vi "Playground_Variant Attributes to Cluster.vi"() -> ()   [LabVIEW 2019]
uses:
  subVIs/typedefs/Schedule Types/Schedule--Ramp.ctl
  Classes/Settings/ObjectSettings/ObjectSettings.lvclass
panel:
  out "Array":variant[](array[variant])
  out "x/y":dbl
  # "Read"
  # "JDP: 4.65363E-5"
  # "JKI: 0.0002399"
  # "Write"
  # "JDP: 3.40146E-5\nJKI: 8.64174E-5"
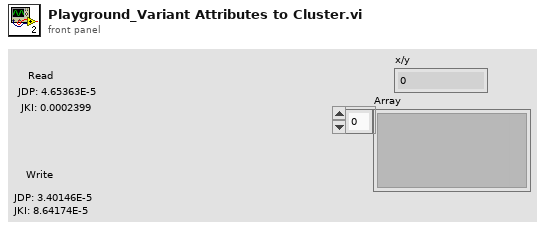
[diagram p1: front panel]
types:
  T1 = typedef "Schedule--Ramp.ctl" = cluster{"Start":dbl, "End":dbl}
  T2 = cluster{"Attribute 1":bool, "Attribute 2":string, "Attribute 3":string}
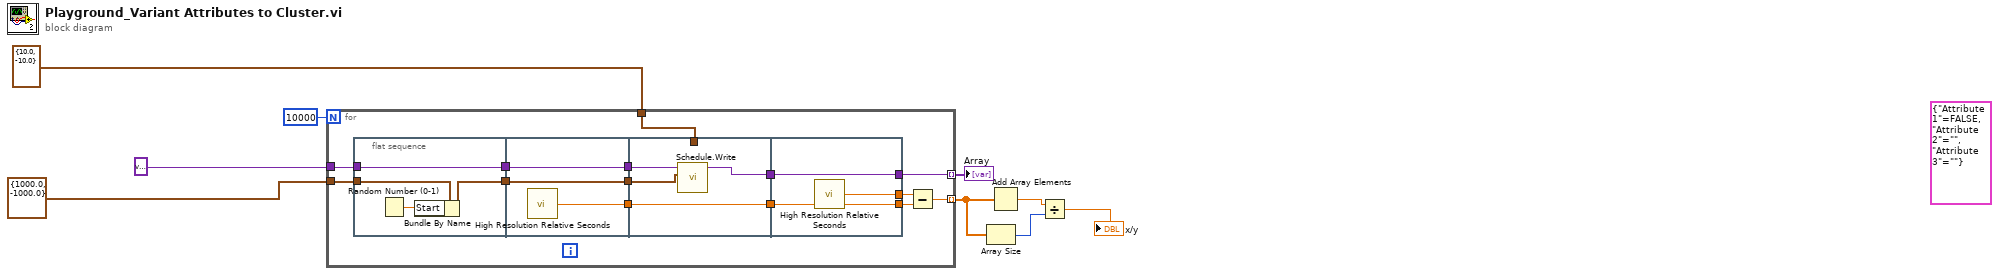
[diagram p0: block diagram]
diagram:
  (unwired) T2 {"Attribute 1"=FALSE, "Attribute 2"="", "Attribute 3"=""}
  n1 = for {
    N: 10000 -> [_]
    tunnel: T1 {"Start"=10.0, "End"=-10.0} ("Ramp") -> [w21]
    tunnel: variant ("LUT In") -> [w23]
    tunnel: [w22] -> w1 mode=indexing
    tunnel: [w14] -> w7 mode=indexing
    tunnel: T1 {"Start"=1000.0, "End"=-1000.0} ("Ramp") -> [w11]
    n2 = flat-sequence {
      tunnel: w23 -> [w27]
      tunnel: [w27] -> w13
      tunnel: [w26] -> w12
      tunnel: w11 -> [w25]
      tunnel: [w30] -> w20
      tunnel: [w29] -> w17
      tunnel: w13 -> [w30]
      tunnel: w12 -> [w28]
      tunnel: [w28] -> w10
      tunnel: w21 -> [_]
      tunnel: w20 -> [w33]
      tunnel: [w32] -> w19
      tunnel: [w34] -> w18
      tunnel: w17 -> [w34]
      tunnel: w10 -> [w31]
      tunnel: [w37] -> w22
      tunnel: w19 -> [w37]
      tunnel: [w36] -> w15
      tunnel: w18 -> [w36]
      tunnel: [w35] -> w16
      frame #0 {
        n3 = Random Number (0-1)() -> (number: 0 to 1=w24:dbl)
        n4 = Bundle By Name(cluster=w25, "Start"=w24) -> (w26:T1)
      }
      frame #1 {
        n5 = call <vilib>:"High Resolution Relative Seconds.vi"() -> ("relative seconds"=w29:dbl)
      }
      frame #2 {
        n6 = call "Schedule.Write.vi"("Data to Write"=w31, "LUT In"=w33) -> ("LUT Out"=w32:variant)  [unwired: 8 in, 1 out]
      }
      frame #3 {
        n7 = call <vilib>:"High Resolution Relative Seconds.vi"() -> ("relative seconds"=w35:dbl)
      }
    }
    n8 = Subtract(x=w16, y=w15) -> (x-y=w14:dbl)
  }
  "Array" <- w1
  n9 = Array Size(array=w7) -> (size(s)=w5:i32)
  n10 = Add Array Elements(numeric array=w7) -> (sum=w6:dbl)
  n11 = Divide(x=w6, y=w5) -> (x/y=→"x/y":dbl)
